vi "XScaleConfigure.vi"(1 "TimeBase":cluster{"Time/Div":dbl} {"Time/Div" scale=5e-06..0.2}) -> (0 "X坐标范围":T1)   [LabVIEW 2012]
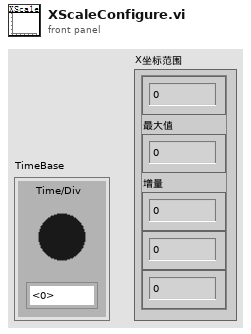
[diagram p1: front panel]
types:
  T1 = cluster{"数值输入控件":dbl, "最大值":dbl, "增量":dbl, "数值输入控件":dbl, "数值输入控件":dbl}
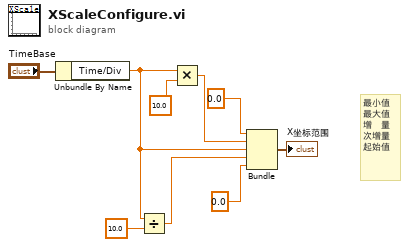
[diagram p0: block diagram]
diagram:
  # "最小值\n最大值\n增   量\n次增量\n起始值"
  n1 = Unbundle By Name("TimeBase") -> ("Time/Div"=w3:dbl)
  n2 = Divide(x=w3, y=10.0) -> (x/y=w6:dbl)
  n3 = Multiply(x=w3, y=10.0) -> (x*y=w1:dbl)
  n4 = Bundle(0.0, w1, "Time/Div"=w3, w6, 0.0) -> (→"X坐标范围":cluster{dbl, dbl, "Time/Div":dbl, dbl, dbl})  [unwired: 1 in]
